vi "bits_to_byte.vi"(2 "error in":errorcluster, 3 "Binary att & channel":string="11111011") -> (0 "error out":errorcluster, 1 "Byte written out":string)   [LabVIEW 2021]
panel:
  out "hex val":string
  out "decimal val":u8
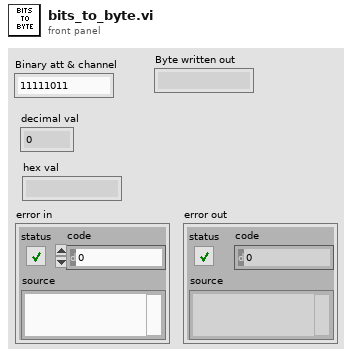
[diagram p1: front panel]
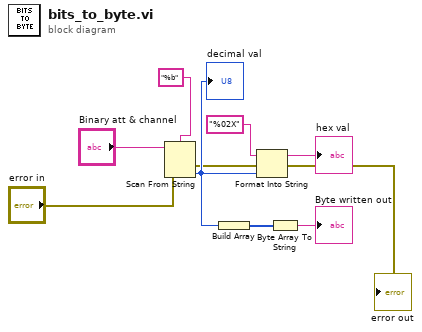
[diagram p0: block diagram]
diagram:
  n1 = Scan From String(format string="%b", input string="Binary att & channel", error in="error in") -> (error out=→"error out":errorcluster, output 1=w5:u8)  [unwired: 2 in, 2 out]
  "decimal val" <- w5
  n2 = Build Array(w5) -> (w4:u8[])
  n3 = Format Into String(format string="%02X", w5) -> (resulting string=→"hex val":string)  [unwired: 2 in, 1 out]
  n4 = Byte Array To String(unsigned byte array=w4) -> (string=→"Byte written out":string)
